vi "getBounds.vi"(0 "reference":refnum<class "GeneralPathEdge.lvclass">, 1 "graphics":refnum<class "Graphics.lvclass">, 5 "error in (no error)":errorcluster) -> (14 "reference out":refnum<class "GeneralPathEdge.lvclass">, 15 "bounds":T1 {"height" format="%.2f"; "width" format="%.2f"; "y" format="%.2f"; "x" format="%.2f"}, 19 "error out":errorcluster)   [LabVIEW 2016, in "GeneralPathEdge.lvclass"]
doc: "public Rectangle2D getBounds(Graphics2D g2)"
uses:
  <resource>/Framework/Providers/Open_GDS/UML/GeneralPathEdge_class/GeneralPathEdge.lvclass
  <resource>/Framework/Providers/Open_GDS/UML/General/Rectangle/Rectangle Rectangle2D.ctl
  <resource>/Framework/Providers/Open_GDS/UML/Graphics_class/Graphics.lvclass
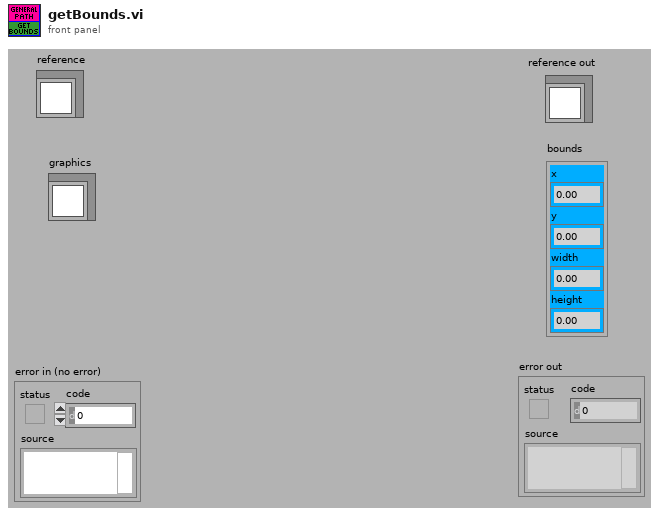
[diagram p1: front panel]
types:
  T1 = typedef "Rectangle Rectangle2D.ctl" = cluster{"x":dbl, "y":dbl, "width":dbl, "height":dbl}
  T2 = typedef "Point Point2D.ctl" = cluster{"x":dbl, "y":dbl}
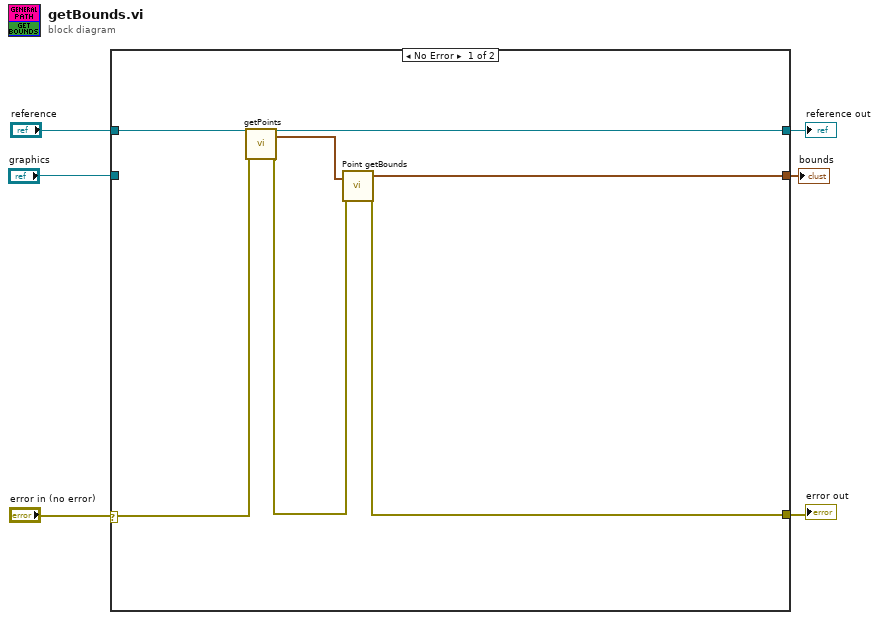
[diagram p0: block diagram]
diagram:
  n1 = case shown="No Error" "error in (no error)" {
    selector: "error in (no error)" -> [w10 w14]
    tunnel: "reference" -> [w13 w15]
    tunnel: [w12 w14] -> w5
    tunnel: [w11 w15] -> w4
    tunnel: [w9 _] -> w2
    tunnel: "graphics" -> [_ _]
    frame No Error {
      n2 = call-dynamic "getPoints.vi"("reference"=w13, "error in (no error)"=w10) -> ("reference out"=w11:refnum<class "GeneralPathEdge.lvclass">, "points"=w8:T2[], "error out"=w7:errorcluster)  [unwired: 15 in]
      n3 = call <resource>:"Point getBounds.vi"("points"=w8, "error in (no error)"=w7) -> ("boundsAdded"=w9:T1, "error out"=w12:errorcluster)  [unwired: 16 out]
    }
    frame Error {
    }
  }
  "reference out" <- w4
  "error out" <- w5
  "bounds" <- w2
